vi "MotorPreMove.vi"(3 "Motor":string="PI1-SHUTTER", 4 "Movement":i32, 9 "error in (no error)":errorcluster) -> (0 "Motor out":string="PI1-SHUTTER", 2 "Go!":refnum<k4>, 6 "error out":errorcluster)   [LabVIEW 2009]
uses:
  Controls/MotorCommand.ctl
  Controls/MotorCommandBasic.ctl
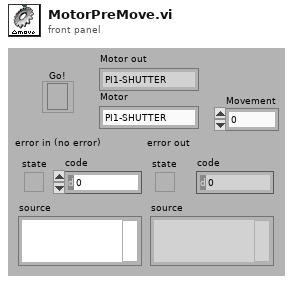
[diagram p1: front panel]
types:
  T1 = typedef "MotorCommandBasic.ctl" = enum16{"SELECT", "MOVE", "PREMOVE", "TURBO", "POS", "NAMED", "INIT", "STOP", "OFF", "SPEED", "QUIT"}
  T2 = typedef "MotorCommand.ctl" = cluster{"Motor":string, "Command":T1, "Movement":i32, "Name":string, "Param":cluster{"VMIN":i32, "VMAX":i32, "ACC":i32}, "Ok?":refnum<k4>, "Go!":refnum<k4>}
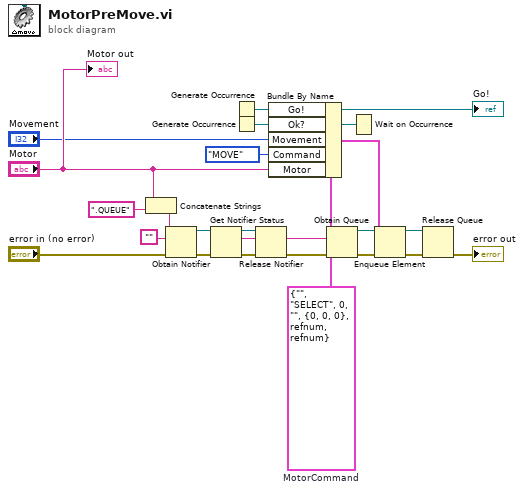
[diagram p0: block diagram]
diagram:
  w20 = T2 {"Motor"="", "Command"=enum."SELECT", "Movement"=0, "Name"="", "Param"={"VMIN"=0, "VMAX"=0, "ACC"=0}, "Ok?"=refnum, "Go!"=refnum}  # MotorCommand
  n1 = Concatenate Strings("Motor", ".QUEUE") -> (w11:string)
  n2 = Obtain Notifier(name (unnamed)=w11, notification data type="", error in (no error)="error in (no error)") -> (notifier out=w12:refnum<notifier>, error out=w13:errorcluster)  [unwired: 1 in, 1 out]
  n3 = Get Notifier Status(notifier=w12, error in (no error)=w13) -> (notifier out=w15:refnum<notifier>, current notification=w8:string, error out=w16:errorcluster)  [unwired: 2 out]
  n4 = Generate Occurrence() -> (w1:refnum<k4>)
  "Go!" <- w1
  n5 = Generate Occurrence() -> (w2:refnum<k4>)
  n6 = Release Notifier(notifier=w15, error in (no error)=w16) -> (error out=w9:errorcluster)  [unwired: 3 out]
  n7 = Bundle By Name(cluster=w20, "Go!"=w1, "Ok?"=w2, "Movement"="Movement", "Command"=MotorCommandBasic."MOVE", "Motor"="Motor") -> (w19:T2)
  n8 = Obtain Queue(name (unnamed)=w8, element data type=w20, error in (no error)=w9) -> (queue out=w22:refnum<queue>, error out=w21:errorcluster)  [unwired: 2 in, 1 out]
  n9 = Wait on Occurrence(2:w2) -> ()  [unwired: 3 out]
  n10 = Enqueue Element(queue=w22, element=w19, error in (no error)=w21) -> (queue out=w17:refnum<queue>, error out=w18:errorcluster)  [unwired: 2 out]
  n11 = Release Queue(queue=w17, error in (no error)=w18) -> (error out=→"error out":errorcluster)  [unwired: 3 out]
  "Motor out" <- "Motor"
